vi "deploy image core.vi"(8 "error in (no error)":errorcluster, 11 "image path":path) -> (0 "error out":errorcluster)   [LabVIEW 2014]
uses:
  <vilib>/Utility/sysdir.llb/System Directory Type.ctl
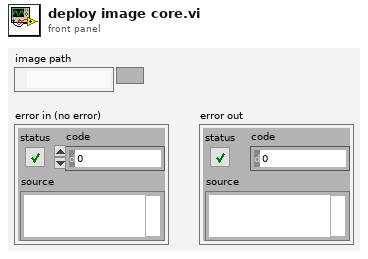
[diagram p1: front panel]
types:
  T1 = typedef "System Directory Type.ctl" = i32
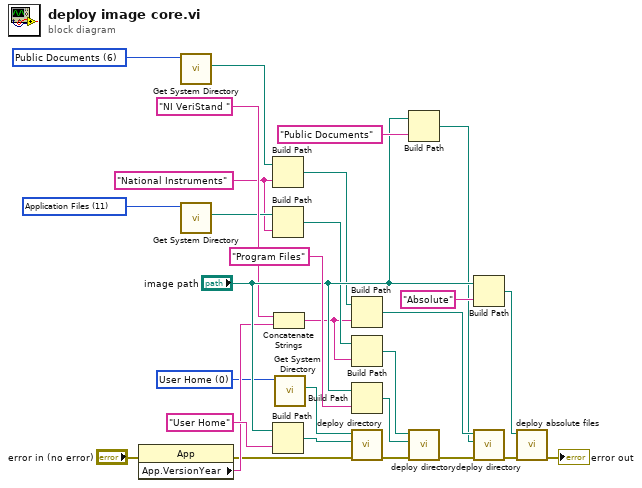
[diagram p0: block diagram]
diagram:
  w14 = T1 0 items=["User Home"=0, "User Desktop"=1, "User Documents"=2, "User Application Data"=3, "User Preferences"=4, "User Temporary"=5, "Public Documents"=6, "Public Application Data"=7, "Public Preferences"=8, "Public Cache"=13, "System Core Libraries"=9, "System Installed Libraries"=10, "Application Files"=11, "Boot Volume Root"=12] ("system directory type")
  w19 = T1 11 items=["User Home"=0, "User Desktop"=1, "User Documents"=2, "User Application Data"=3, "User Preferences"=4, "User Temporary"=5, "Public Documents"=6, "Public Application Data"=7, "Public Preferences"=8, "Public Cache"=13, "System Core Libraries"=9, "System Installed Libraries"=10, "Application Files"=11, "Boot Volume Root"=12] ("system directory type")
  w15 = "National Instruments"
  w24 = T1 6 items=["User Home"=0, "User Desktop"=1, "User Documents"=2, "User Application Data"=3, "User Preferences"=4, "User Temporary"=5, "Public Documents"=6, "Public Application Data"=7, "Public Preferences"=8, "Public Cache"=13, "System Core Libraries"=9, "System Installed Libraries"=10, "Application Files"=11, "Boot Volume Root"=12] ("system directory type")
  n1 = property class="App"(error in="error in (no error)") -> (error out=w10:errorcluster, "App.VersionYear"=w21:string)  [unwired: 1 in, 1 out]
  n2 = call <vilib>:"Get System Directory.vi"("system directory type"=w24) -> ("system directory"=w23:path)  [unwired: 10 in]
  n3 = call <vilib>:"Get System Directory.vi"("system directory type"=w19) -> ("system directory"=w18:path)  [unwired: 10 in]
  n4 = Build Path(base path=w23, name or relative path=w15) -> (appended path=w22:path)
  n5 = Build Path(base path=w18, name or relative path=w15) -> (appended path=w17:path)
  n6 = Build Path(base path="image path", name or relative path="User Home") -> (appended path=w11:path)
  n7 = Concatenate Strings("NI VeriStand ", w21) -> (w16:string)
  n8 = call <vilib>:"Get System Directory.vi"("system directory type"=w14) -> ("system directory"=w12:path)  [unwired: 10 in]
  n9 = Build Path(base path=w22, name or relative path=w16) -> (appended path=w5:path)
  n10 = Build Path(base path=w17, name or relative path=w16) -> (appended path=w6:path)
  n11 = Build Path(base path="image path", name or relative path="Program Files") -> (appended path=w7:path)
  n12 = call "deploy directory.vi"("error in (no error)"=w10, "from path"=w11, "to path"=w12) -> ("error out"=w9:errorcluster)  [unwired: 8 in]
  n13 = Build Path(base path="image path", name or relative path="Public Documents") -> (appended path=w4:path)
  n14 = call "deploy directory.vi"("error in (no error)"=w9, "from path"=w7, "to path"=w6) -> ("error out"=w8:errorcluster)  [unwired: 8 in]
  n15 = Build Path(base path="image path", name or relative path="Absolute") -> (appended path=w2:path)
  n16 = call "deploy directory.vi"("error in (no error)"=w8, "from path"=w4, "to path"=w5) -> ("error out"=w3:errorcluster)  [unwired: 8 in]
  n17 = call "deploy absolute files.vi"("error in (no error)"=w3, "appended path"=w2) -> ("error out"=→"error out":errorcluster)  [unwired: 9 in]
